vi "ReadWrite.ProcessData.Reset.vi"(8 "error in":errorcluster, 10 "timeout ms":i32=100, 11 "ReadWrite in":refnum<class "ReadWrite.lvclass">) -> (0 "error out":errorcluster, 1 "Timeout?":bool, 3 "ReadWrite out":refnum<class "ReadWrite.lvclass">)   [LabVIEW 2024, in "VS Plugin Data Access Engine.lvlib" / "ReadWrite.lvclass"]
uses:
  ReadWrite.lvclass
  ReadWrite.lvclass/ReadWrite.ctl
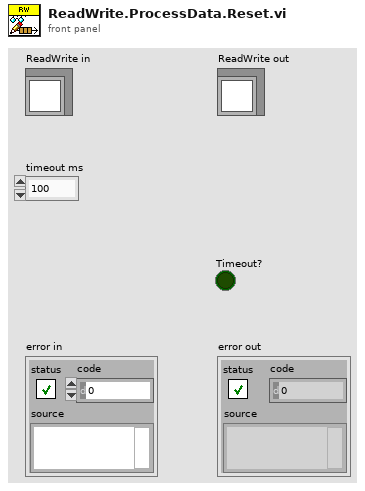
[diagram p1: front panel]
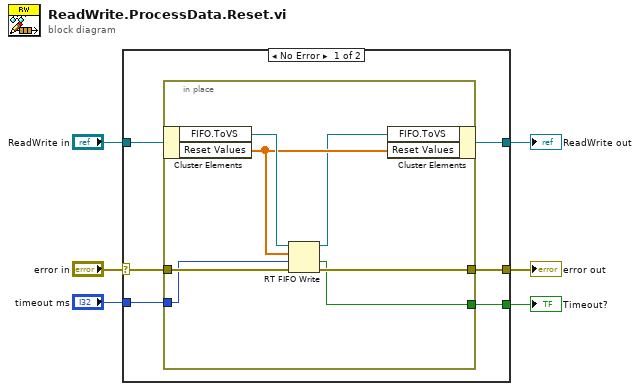
[diagram p0: block diagram]
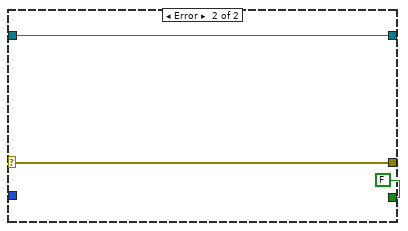
[diagram p2: hidden frame]
diagram:
  n1 = case shown="No Error" "error in" {
    selector: "error in" -> [w12 w22]
    tunnel: [w11 w22] -> w5
    tunnel: [w9 w20] -> w1
    tunnel: "ReadWrite in" -> [w10 w20]
    tunnel: "timeout ms" -> [w8 _]
    tunnel: [w7 FALSE ("empty?")] -> w3
    frame No Error {
      n2 = in-place {
        in-place-border: w12 -> [w18]
        in-place-border: [w19] -> w11
        in-place-border: w8 -> [w13]
        in-place-border: [w14] -> w7
        n3 = in-place-cluster #1(w10) -> ("FIFO.ToVS"=w17:refnum<k33>, "Reset Values"=w16:dbl[])
        n4 = RT FIFO Write(0:w17, 1:w16, 2:w13, 3:w18) -> (8:w15:refnum<k33>, 10:w14:bool, 11:w19:errorcluster)  [unwired: 1 in, 1 out]
        n5 = in-place-cluster #1("FIFO.ToVS"=w15, "Reset Values"=w16) -> (w9:refnum<class "ReadWrite.lvclass">)
      }
    }
    frame Error {
    }
  }
  "error out" <- w5
  "ReadWrite out" <- w1
  "Timeout?" <- w3
